vi "Toggle.vi"(9 "Input":bool) -> (1 "Toggled output":bool)   [LabVIEW 2015]
doc: "Outputs toggles when a rising edge is detected"
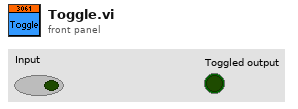
[diagram p1: front panel]
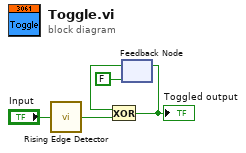
[diagram p0: block diagram]
diagram:
  n1 = call "Rising Edge Detector.vi"("Input"="Input") -> ("Rising edge?"=w3:bool)
  n2 = feedback #1(FALSE) -> (w2:bool)
  n3 = Exclusive Or(1:w3, 2:w2) -> (0:w4:bool)
  "Toggled output" <- w4
  n4 = feedback-in #1(w4) -> ()
